vi "Limiting.vi"(9 "Maximum":dbl, 10 "Value":dbl, 11 "Minimum":dbl) -> (3 "Output":i16)   [LabVIEW 2018, in "Pid.lvlib"]
uses:
  Pid.lvlib
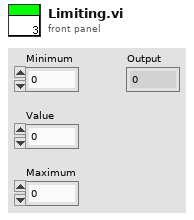
[diagram p1: front panel]
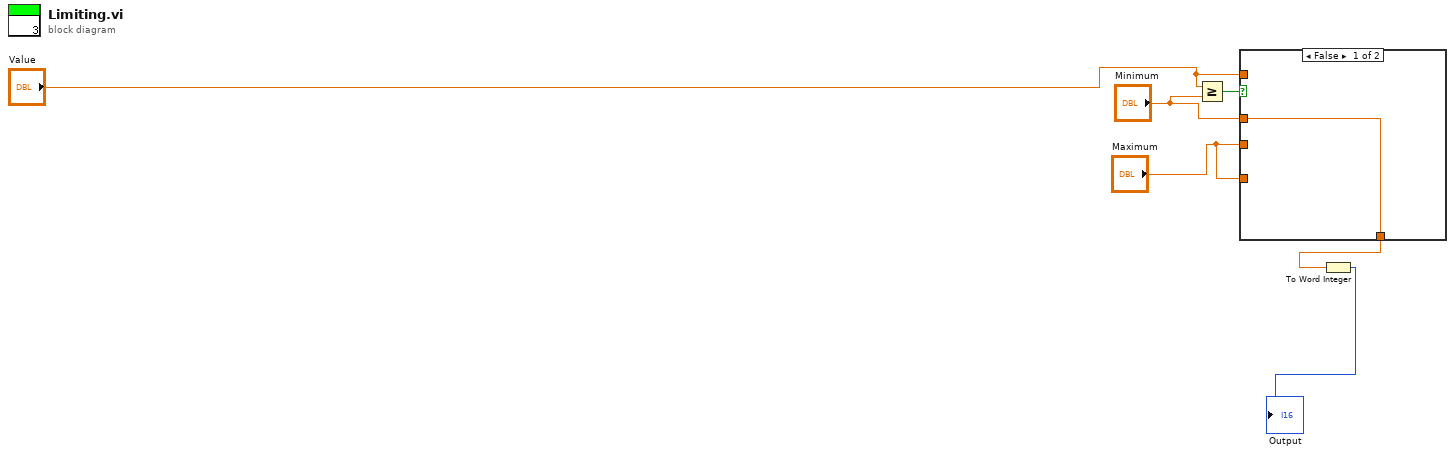
[diagram p0: block diagram]
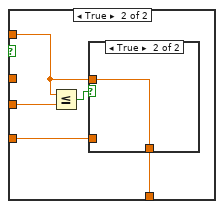
[diagram p2: hidden frame]
diagram:
  n1 = Greater Or Equal?(x="Value", y="Minimum") -> (x >= y?=w1:bool)
  n2 = case shown="False" w1 {
    tunnel: "Value" -> [_ w10]
    tunnel: "Maximum" -> [_ w12]
    tunnel: [w7 w9] -> w3
    tunnel: "Maximum" -> [_ w8]
    tunnel: "Minimum" -> [w7 _]
    frame False {
    }
    frame True {
      n3 = Less Or Equal?(x=w10, y=w12) -> (x <= y?=w11:bool)
      n4 = case shown="True" w11 {
        tunnel: w10 -> [_ w14]
        tunnel: [w13 w14] -> w9
        tunnel: w8 -> [w13 _]
        frame False {
        }
        frame True {
        }
      }
    }
  }
  n5 = To Word Integer(number=w3) -> (16bit integer=→"Output":i16)
